vi "Test Serialize Variant Attributes.vi"(8 "error in (no error)":errorcluster) -> (0 "error out":errorcluster)   [LabVIEW 2015]
uses:
  src/Serializer/JSON Serializer/JSON Serializer.lvclass
  <vilib>/addons/_JKI Toolkits/Caraya/classes/Test/Test.lvclass
  <vilib>/addons/_JKI Toolkits/Caraya/classes/Assert/Assert.lvclass
panel:
  out "String 4":string
  out "String 3":string
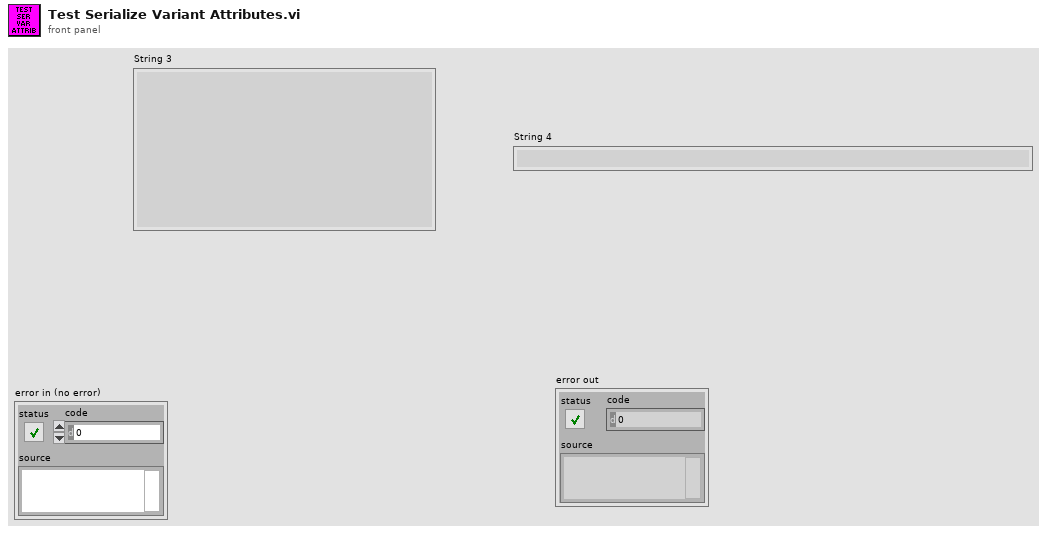
[diagram p1: front panel]
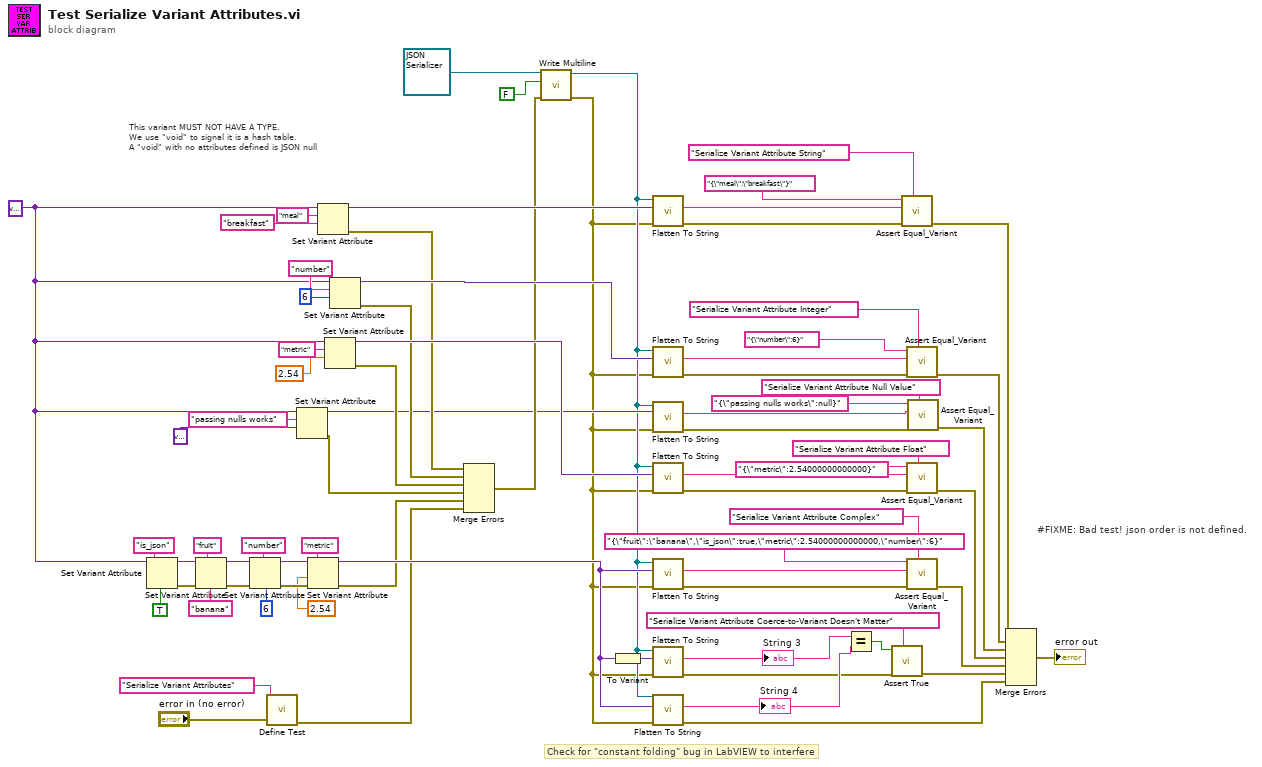
[diagram p0: block diagram]
diagram:
  w12 = variant
  # "#FIXME: Bad test! json order is not defined."
  # "This variant MUST NOT HAVE A TYPE.\nWe use \"void\" to signal it is a hash table.\nA \"void\" with no attributes defined is JSON null"
  # "Check for \"constant folding\" bug in LabVIEW to interfere"
  n1 = Set Variant Attribute(Variant=w12, name="is_json", value=TRUE) -> (Variant out=w44:variant, error out=w75:errorcluster)  [unwired: 1 in, 1 out]
  n2 = Set Variant Attribute(Variant=w44, name="fruit", value="banana" ("name"), error in=w75) -> (Variant out=w43:variant, error out=w74:errorcluster)  [unwired: 1 out]
  n3 = Set Variant Attribute(Variant=w43, name="number", value=6, error in=w74) -> (Variant out=w42:variant, error out=w73:errorcluster)  [unwired: 1 out]
  n4 = call <vilib>:"Define Test.vi"("error in (no error)"="error in (no error)", "Label (VI Title)"="Serialize Variant Attributes") -> ("error out"=w14:errorcluster)  [unwired: 9 in]
  n5 = Set Variant Attribute(Variant=w12, name="passing nulls works", value=variant) -> (Variant out=w7:variant, error out=w10:errorcluster)  [unwired: 1 in, 1 out]
  n6 = Set Variant Attribute(Variant=w42, name="metric", value=2.54, error in=w73) -> (Variant out=w24:variant, error out=w15:errorcluster)  [unwired: 1 out]
  n7 = Set Variant Attribute(Variant=w12, name="meal", value="breakfast" ("name")) -> (Variant out=w41:variant, error out=w29:errorcluster)  [unwired: 1 in, 1 out]
  n8 = Set Variant Attribute(Variant=w12, name="metric", value=2.54) -> (Variant out=w36:variant, error out=w27:errorcluster)  [unwired: 1 in, 1 out]
  n9 = Set Variant Attribute(Variant=w12, name="number", value=6) -> (Variant out=w40:variant, error out=w28:errorcluster)  [unwired: 1 in, 1 out]
  n10 = Merge Errors(w29, w28, w27, w10, w15, w14) -> (w23:errorcluster)
  n11 = call-dynamic "Write Multiline.vi"("error in (no error)"=w23, "Multiline"=FALSE, "JSON Serializer in"=refnum<class "JSON Serializer.lvclass"> refnum ("JKI JSON Serialization.lvlib:JSON Serializer.lvclass")) -> ("error out"=w5:errorcluster, "JSON Serializer out"=w6:refnum<class "JSON Serializer.lvclass">)  [unwired: 7 in]
  n12 = To Variant(anything=w24) -> (Variant=w39:variant)
  n13 = call-dynamic "Flatten To String.vi"("error in (no error)"=w5, "Variant"=w41, "JSON Serializer in"=w6) -> ("error out"=w66:errorcluster, "String"=w64:string)  [unwired: 6 in, 1 out]
  n14 = call-dynamic "Flatten To String.vi"("error in (no error)"=w5, "Variant"=w40, "JSON Serializer in"=w6) -> ("error out"=w60:errorcluster, "String"=w59:string)  [unwired: 6 in, 1 out]
  n15 = call-dynamic "Flatten To String.vi"("error in (no error)"=w5, "Variant"=w7, "JSON Serializer in"=w6) -> ("error out"=w4:errorcluster, "String"=w2:string)  [unwired: 6 in, 1 out]
  n16 = call-dynamic "Flatten To String.vi"("error in (no error)"=w5, "Variant"=w36, "JSON Serializer in"=w6) -> ("error out"=w61:errorcluster, "String"=w18:string)  [unwired: 6 in, 1 out]
  n17 = call-dynamic "Flatten To String.vi"("error in (no error)"=w5, "Variant"=w24, "JSON Serializer in"=w6) -> ("error out"=w26:errorcluster, "String"=w22:string)  [unwired: 6 in, 1 out]
  n18 = call-dynamic "Flatten To String.vi"("error in (no error)"=w5, "Variant"=w39, "JSON Serializer in"=w6) -> ("error out"=w32:errorcluster, "String"=w35:string)  [unwired: 6 in, 1 out]
  "String 3" <- w35
  n19 = call-dynamic "Flatten To String.vi"("error in (no error)"=w5, "Variant"=w24, "JSON Serializer in"=w6) -> ("error out"=w21:errorcluster, "String"=w34:string)  [unwired: 6 in, 1 out]
  "String 4" <- w34
  n20 = Equal?(x=w35, y=w34) -> (x = y?=w33:bool)
  n21 = call <vilib>:"Assert True.vi"("Label"="Serialize Variant Attribute Coerce-to-Variant Doesn't Matter", "error in (no error)"=w32, "True?"=w33) -> ("error out"=w20:errorcluster)  [unwired: 8 in]
  n22 = call <vilib>:"Assert Equal_Variant.vi"("Label"="Serialize Variant Attribute String", "error in (no error)"=w66, "Y"=w64, "X"="{\"meal\":\"breakfast\"}" ("String 2")) -> ("error out"=w63:errorcluster)  [unwired: 7 in]
  n23 = call <vilib>:"Assert Equal_Variant.vi"("Label"="Serialize Variant Attribute Integer", "error in (no error)"=w60, "Y"=w59, "X"="{\"number\":6}" ("String")) -> ("error out"=w9:errorcluster)  [unwired: 7 in]
  n24 = call <vilib>:"Assert Equal_Variant.vi"("Label"="Serialize Variant Attribute Float", "error in (no error)"=w61, "Y"=w18, "X"="{\"metric\":2.54000000000000}" ("String 2")) -> ("error out"=w67:errorcluster)  [unwired: 7 in]
  n25 = call <vilib>:"Assert Equal_Variant.vi"("Label"="Serialize Variant Attribute Complex", "error in (no error)"=w26, "Y"=w22, "X"="{\"fruit\":\"banana\",\"is_json\":true,\"metric\":2.54000000000000,\"number\":6}" ("String")) -> ("error out"=w19:errorcluster)  [unwired: 7 in]
  n26 = call <vilib>:"Assert Equal_Variant.vi"("Label"="Serialize Variant Attribute Null Value", "error in (no error)"=w4, "Y"=w2, "X"="{\"passing nulls works\":null}" ("String")) -> ("error out"=w8:errorcluster)  [unwired: 7 in]
  n27 = Merge Errors(w63, w9, w8, w67, w19, w20, w21) -> (→"error out":errorcluster)
